vi "NIMS_DF_fir_linf(n, f, mag, w, ftype, t).vi"(6 "t":T1(ring), 7 "ftype":string, 8 "w":dbl[](array[numeric]), 9 "mag":dbl[](array[numeric]), 10 "f":dbl[](array[numeric]), 11 "n":i32=20) -> (0 "error":i32, 3 "b":dbl[](array[numeric]))   [LabVIEW 2017, in "NI_DigFilter_MathScript.lvlib"]
uses:
  <vilib>/addons/Digital Filter Design/NI_DigFilter_MathScript.lvlib
  <vilib>/addons/Digital Filter Design/_REMEZ.llb/remez_fir filter type.ctl
  <vilib>/addons/Digital Filter Design/NI_DigFilterLicensed.lvlib
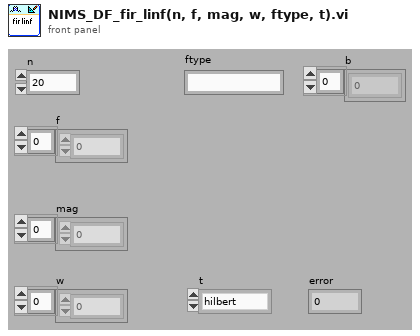
[diagram p1: front panel]
types:
  T1 = enum32{"hilbert", "differentiator", "minphase", "maxphase"}
  T2 = typedef "NI_DigFilterLicensed.lvlib/remez_fir filter type.ctl" = enum32{"Symmetric", "Antisymmetric", "Differentiator", "Hilbert", "Minimum Phase", "Maximum Phase"}
  T3 = typedef "NI_DigFilterLicensed.lvlib/DFD Adv Band Spec.ctl" = cluster{"band specification":cluster{"freq":dbl, "amplitude":dbl, "weight":dbl}[], "ripple constraint":dbl}
  T4 = typedef "NI_DigFilterLicensed.lvlib/DFD Filter Obj.ctl" = cluster{"mSRate_Fs":dbl, "mSRate_Version":string, "mSRate_Comments":string, "mSRate_OrgCoef":T5, "mSRate_CurCoef":T5, "mSRate_Quantized?":bool, "mSRate_QCoef":T5, "mSRate_QSettings":T7[], "mSRate_Order":i32, "mSRate_Scaling":cluster{"mSRate_ScaleByPowerOf2?":bool, "mSRate_ScaleType":T9}}
  T5 = typedef "NI_DigFilterLicensed.lvlib/DFD Filter Coef.ctl" = cluster{"type":T6, "gain":dbl, "coef a (k)":dbl[], "coef b (v)":dbl[]}
  T6 = typedef "NI_DigFilterLicensed.lvlib/DFD Filter Structure Type Selector.ctl" = enum16{"Undefined", "FIR Direct Form", "FIR Direct Form Transposed", "FIR Symmetric", "FIR Antisymmetric", "IIR Direct Form I", "IIR Direct Form I Transposed", "IIR Direct Form II", "IIR Direct Form II Transposed", "IIR Cascaded Second Order Sections Form I", "IIR Cascaded Second Order Sections Form I Transposed", "IIR Cascaded Second Order Sections Form II", "IIR Cascaded Second Order Sections Form II Transposed", "Lattice Allpass (basic sections)", "Lattice Allpass (one multiplier sections)", "Lattice Allpass (normalized sections)", "Lattice AR (basic sections)", "Lattice AR (one multiplier sections)", "Lattice AR (normalized sections)", "Lattice MA (minimum phase)", "Lattice MA (maximum phase)", "Lattice ARMA (basic sections)", "Lattice ARMA (one multiplier sections)", "Lattice ARMA (normalized sections)"}
  T7 = typedef "NI_DigFilterLicensed.lvlib/dfd_Internal Quantization Settings.ctl" = cluster{"source":T8, "wl":i16, "iwl":i16, "overflow mode":enum16{"Saturation", "Wrap"}, "rounding mode":enum16{"Nearest", "Truncation"}, "signed?":bool}
  T8 = typedef "NI_DigFilterLicensed.lvlib/dfd_Internal Quantization Srcs.ctl" = u16
  T9 = typedef "NI_DigFilterLicensed.lvlib/DFD Coef Norm Type.ctl" = enum16{"No Norm", "Time Domain 1-Norm", "Time Domain 2-Norm", "Time Domain Inf-Norm"}
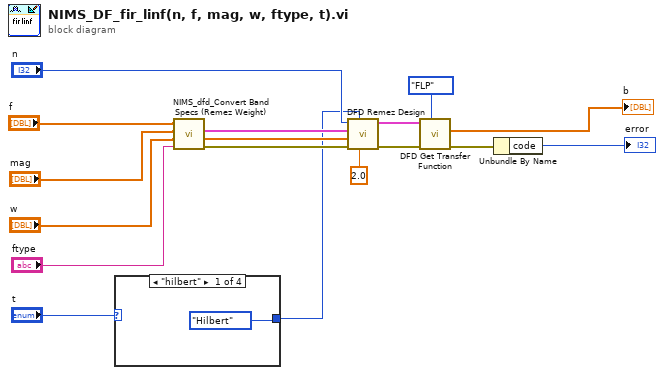
[diagram p0: block diagram]
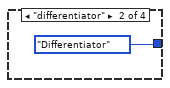
[diagram p2: hidden frame]
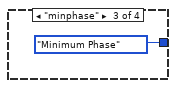
[diagram p3: hidden frame]
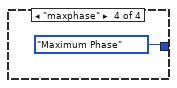
[diagram p4: hidden frame]
diagram:
  n1 = case shown="\"hilbert\"" "t" {
    tunnel: [remez_fir_filter_type."Hilbert" ("filter type") remez_fir_filter_type."Differentiator" ("filter type") remez_fir_filter_type."Minimum Phase" ("filter type") remez_fir_filter_type."Maximum Phase" ("filter type")] -> w2
    frame "hilbert" {
    }
    frame "differentiator" {
    }
    frame "minphase" {
    }
    frame "maxphase" {
    }
  }
  n2 = call <vilib>:"NIMS_dfd_Convert Band Specs (Remez Weight).vi"("s"="ftype", "Weight"="w", "A"="mag", "F"="f") -> ("error out"=w6:errorcluster, "freqs of exact gain [Hz]"=w5:dbl[], "band specs"=w7:T3[])  [unwired: 5 out]
  n3 = call <vilib>:"DFD Remez Design.vi"("fs [Hz]"=2.0, "filter type"=w2, "error in (no error)"=w6, "freqs of exact gain [Hz]"=w5, "band specs"=w7, "order"="n") -> ("error out"=w13:errorcluster, "filter out"=w14:T4)  [unwired: 1 in, 3 out]
  n4 = call <vilib>:"DFD Get Transfer Function.vi"("type (FLP)"=enum16{"FLP", "FXP"}."FLP", "error in (no error)"=w13, "filter in"=w14) -> ("error out"=w17:errorcluster, "numerator"=→"b":dbl[])  [unwired: 7 out]
  n5 = Unbundle By Name(w17) -> ("code"=→"error":i32)
